vi "Przyklad maszyna stanow Bartczak.vi"() -> ()   [LabVIEW 2023]
uses:
  <vilib>/Utility/file.llb/Write Delimited Spreadsheet (DBL).vi
panel:
  in  "OK Button 2":bool
  in  "Numeric":u32
  out "Waveform Graph":dbl[](graph)
  out "Enum":enum16{"wait", "measure"}(ring)
  out ".not. x?":bool
  in  "OK Button":bool
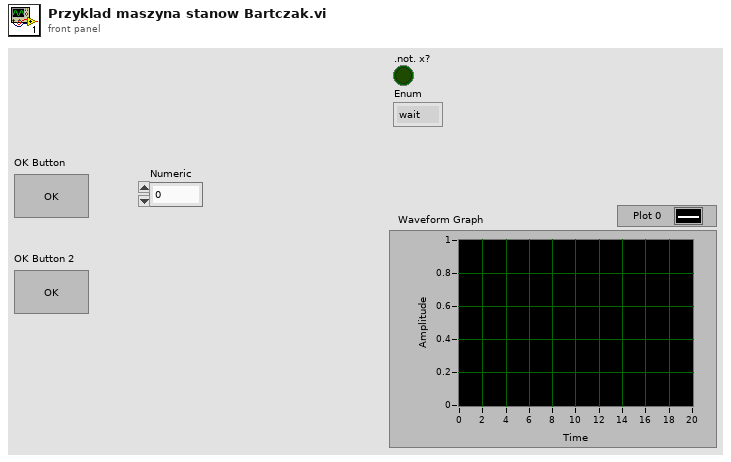
[diagram p1: front panel]
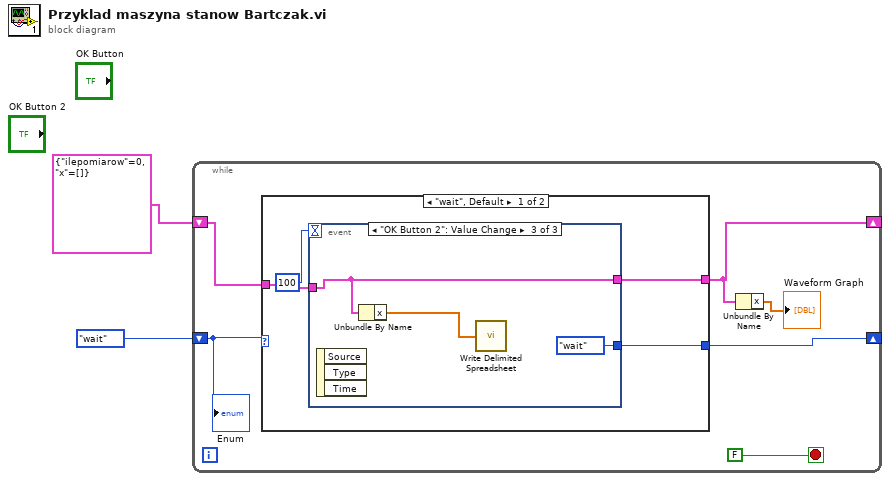
[diagram p0: block diagram]
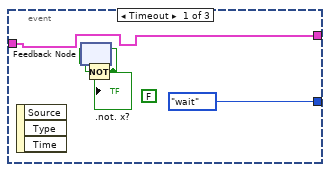
[diagram p2: hidden frame]
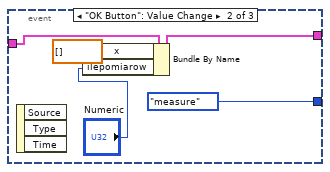
[diagram p3: hidden frame]
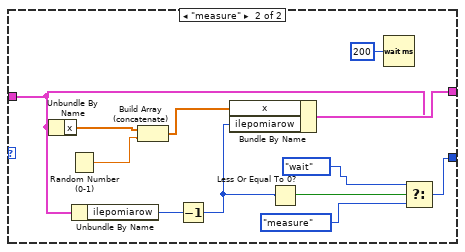
[diagram p4: hidden frame]
diagram:
  n1 = while {
    shift-right: [w7] -> _
    shift-left: enum16{"wait", "measure"}."wait" -> [w8]
    shift-right: [w4] -> _
    shift-left: cluster{"ilepomiarow":u32, "x":dbl[]} {"ilepomiarow"=0, "x"=[]} -> [w5]
    stop <- FALSE stop-if-true
    n2 = case shown="\"wait\", Default" w8 {
      tunnel: [w12 w26] -> w7
      tunnel: [w10 w34] -> w4
      tunnel: w5 -> [w9 w32]
      frame "wait", Default {
        n3 = event shown="[2] \"OK Button 2\": Value Change" {
          selector: _ -> [_ _ _]
          dyn-events: _ -> [_ _ _]
          timeout: 100 -> [_ _ _]
          tunnel: [enum16{"wait", "measure"}."wait" enum16{"wait", "measure"}."measure" enum16{"wait", "measure"}."wait"] -> w12
          tunnel: [w13 w19 w23] -> w10
          tunnel: w9 -> [w13 w20 w23]
          event Timeout {
            (unwired) FALSE (".not. x?")
            n4 = event-data() -> ()  [unwired: 1 in, 3 out]
            n5 = feedback #1() -> (w14:bool)  [unwired: 1 in]
            n6 = Not(x=w14) -> (.not. x?=w15:bool)
            ".not. x?" <- w15
            n7 = feedback-in #1(w15) -> ()
          }
          event "OK Button": Value Change {
            n8 = event-data() -> ()  [unwired: 1 in, 3 out]
            n9 = Bundle By Name(cluster=w20, "x"=dbl[] [], "ilepomiarow"="Numeric") -> (w19:cluster{"ilepomiarow":u32, "x":dbl[]})
          }
          event "OK Button 2": Value Change {
            n10 = event-data() -> ()  [unwired: 1 in, 3 out]
            n11 = Unbundle By Name(w23) -> ("x"=w22:dbl[])
            n12 = call-poly <vilib>:"Write Delimited Spreadsheet.vi"("1D data"=w22) -> ()  [unwired: 13 in, 2 out]
          }
        }
      }
      frame "measure" {
        n13 = Unbundle By Name(w32) -> ("x"=w36:dbl[])
        n14 = Random Number (0-1)() -> (number: 0 to 1=w35:dbl)
        n15 = Unbundle By Name(w32) -> ("ilepomiarow"=w31:u32)
        n16 = Build Array (concatenate)(w36, w35) -> (w33:dbl[])
        n17 = Decrement(x=w31) -> (x-1=w30:u32)
        n18 = Bundle By Name(cluster=w32, "x"=w33, "ilepomiarow"=w30) -> (w34:cluster{"ilepomiarow":u32, "x":dbl[]})
        n19 = Less Or Equal To 0?(x=w30) -> (x <= 0?=w29:bool)
        n20 = Wait (ms)(milliseconds to wait=u32 200) -> ()  [unwired: 1 out]
        n21 = Select(t=enum16{"wait", "measure"}."wait", s=w29, f=enum16{"wait", "measure"}."measure") -> (s? t:f=w26:enum16{"wait", "measure"})
      }
    }
    n22 = Unbundle By Name(w4) -> ("x"=→"Waveform Graph":dbl[])
    "Enum" <- w8
  }
